vi "JV Measurement.vi"(9 "Max (V)":dbl=1.4, 11 "Step (V)":dbl=0.01) -> ()   [LabVIEW 2011]
uses:
  <instrlib>/keithley_24xx/Keithley 24XX/Public/Data/Read (Single Point).vi
  <instrlib>/keithley_24xx/Keithley 24XX/Keithley 24XX.lvlib
panel:
  in  "Variable Value":string="x"
  in  "Variable":string="x"
  in  "Tab Control":enum32{"J-V Scan", "J-t Scan"}(tab)
  in  "Min (V)":dbl
  in  "Stabilisation mode":enum16{"Voltage", "Current"}(ring)
  in  "Stabilisation time (s)":dbl=5.0
  in  "Stabilisation level \n(A or V depending on mode)":dbl=1.4
  in  "Device Area (cm^2)":dbl=0.12
  in  "Measurement Delay (ms)":dbl=10.0
  in  "Initial scan direction":bool=TRUE
  in  "Device Structure":bool
  in  "J-V Scan":bool
  in  "Exit Program":bool
  in  "Device Structure":bool
  in  "Initial scan direction":bool=TRUE
  in  "Measurement Delay (ms)":dbl=100.0
  in  "Device Area (cm^2)":dbl=0.12
  in  "Min (V)":dbl
  in  "Max (V)":dbl=1.4
  in  "Step Voltage (V)":dbl=0.1
  in  "J-t Scan":bool
  in  "Step time (s)":dbl=1.0
  in  "Integration time":enum16{"Fast", "Normal", "High Accuracy"}(ring)
  in  "Pixel":string(combo)="1"
  in  "Condition":string(combo)="Light"
  in  "Compliance  Level":dbl=0.1
  out "Log Table":string[][](table)
  out "JV Curve":cluster{"Y":dbl[], "Y":dbl[]}[](graph)
  in  "Sample Name":string
  in  "Experiment Title":string
  in  "User Name":string
  # "Label"
  # "Pixel"
  # "Condition"
  # "Jsc"
  # "Voc"
  # "PCE"
  # "FF"
  # "Vmp"
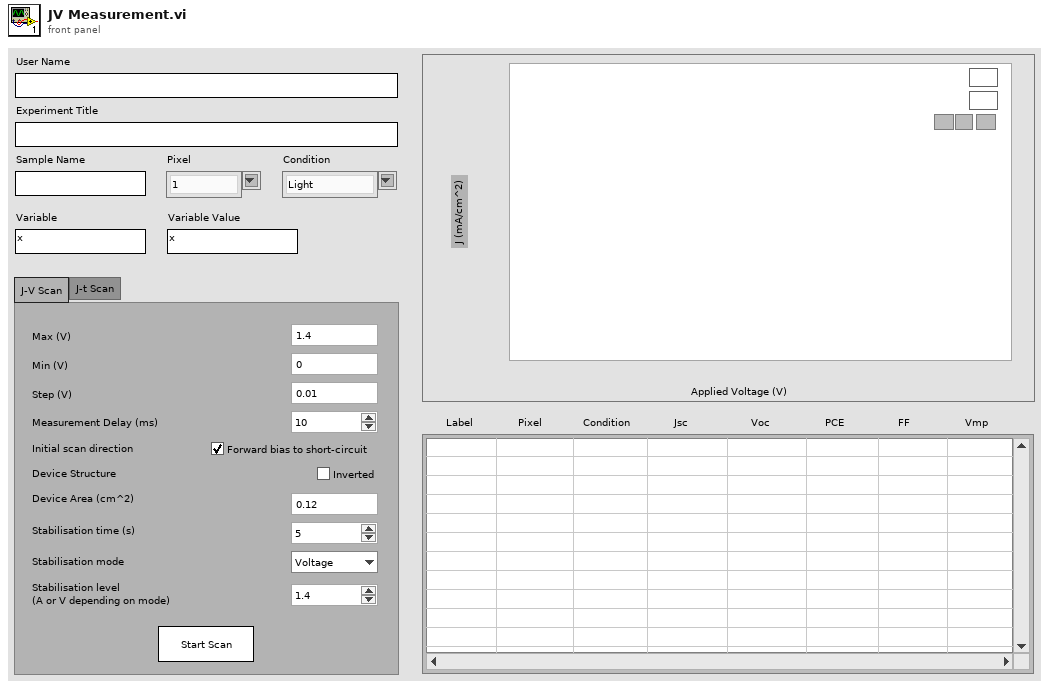
[diagram p1: front panel]
types:
  T1 = cluster{"Cell position":i32, "Cell Label":string, "Pixel":i32, "Area":dbl, "Variable":string, "Variable Value":string, "Scan settings in queue":u16, "Light or dark":string}
  T2 = typedef "imagedata.ctl" = cluster{"image type":i32, "image depth":i32, "image":u8[], "mask":u8[], "colors":u32[], "Rectangle":cluster{"left":i16, "top":i16, "right":i16, "bottom":i16}}
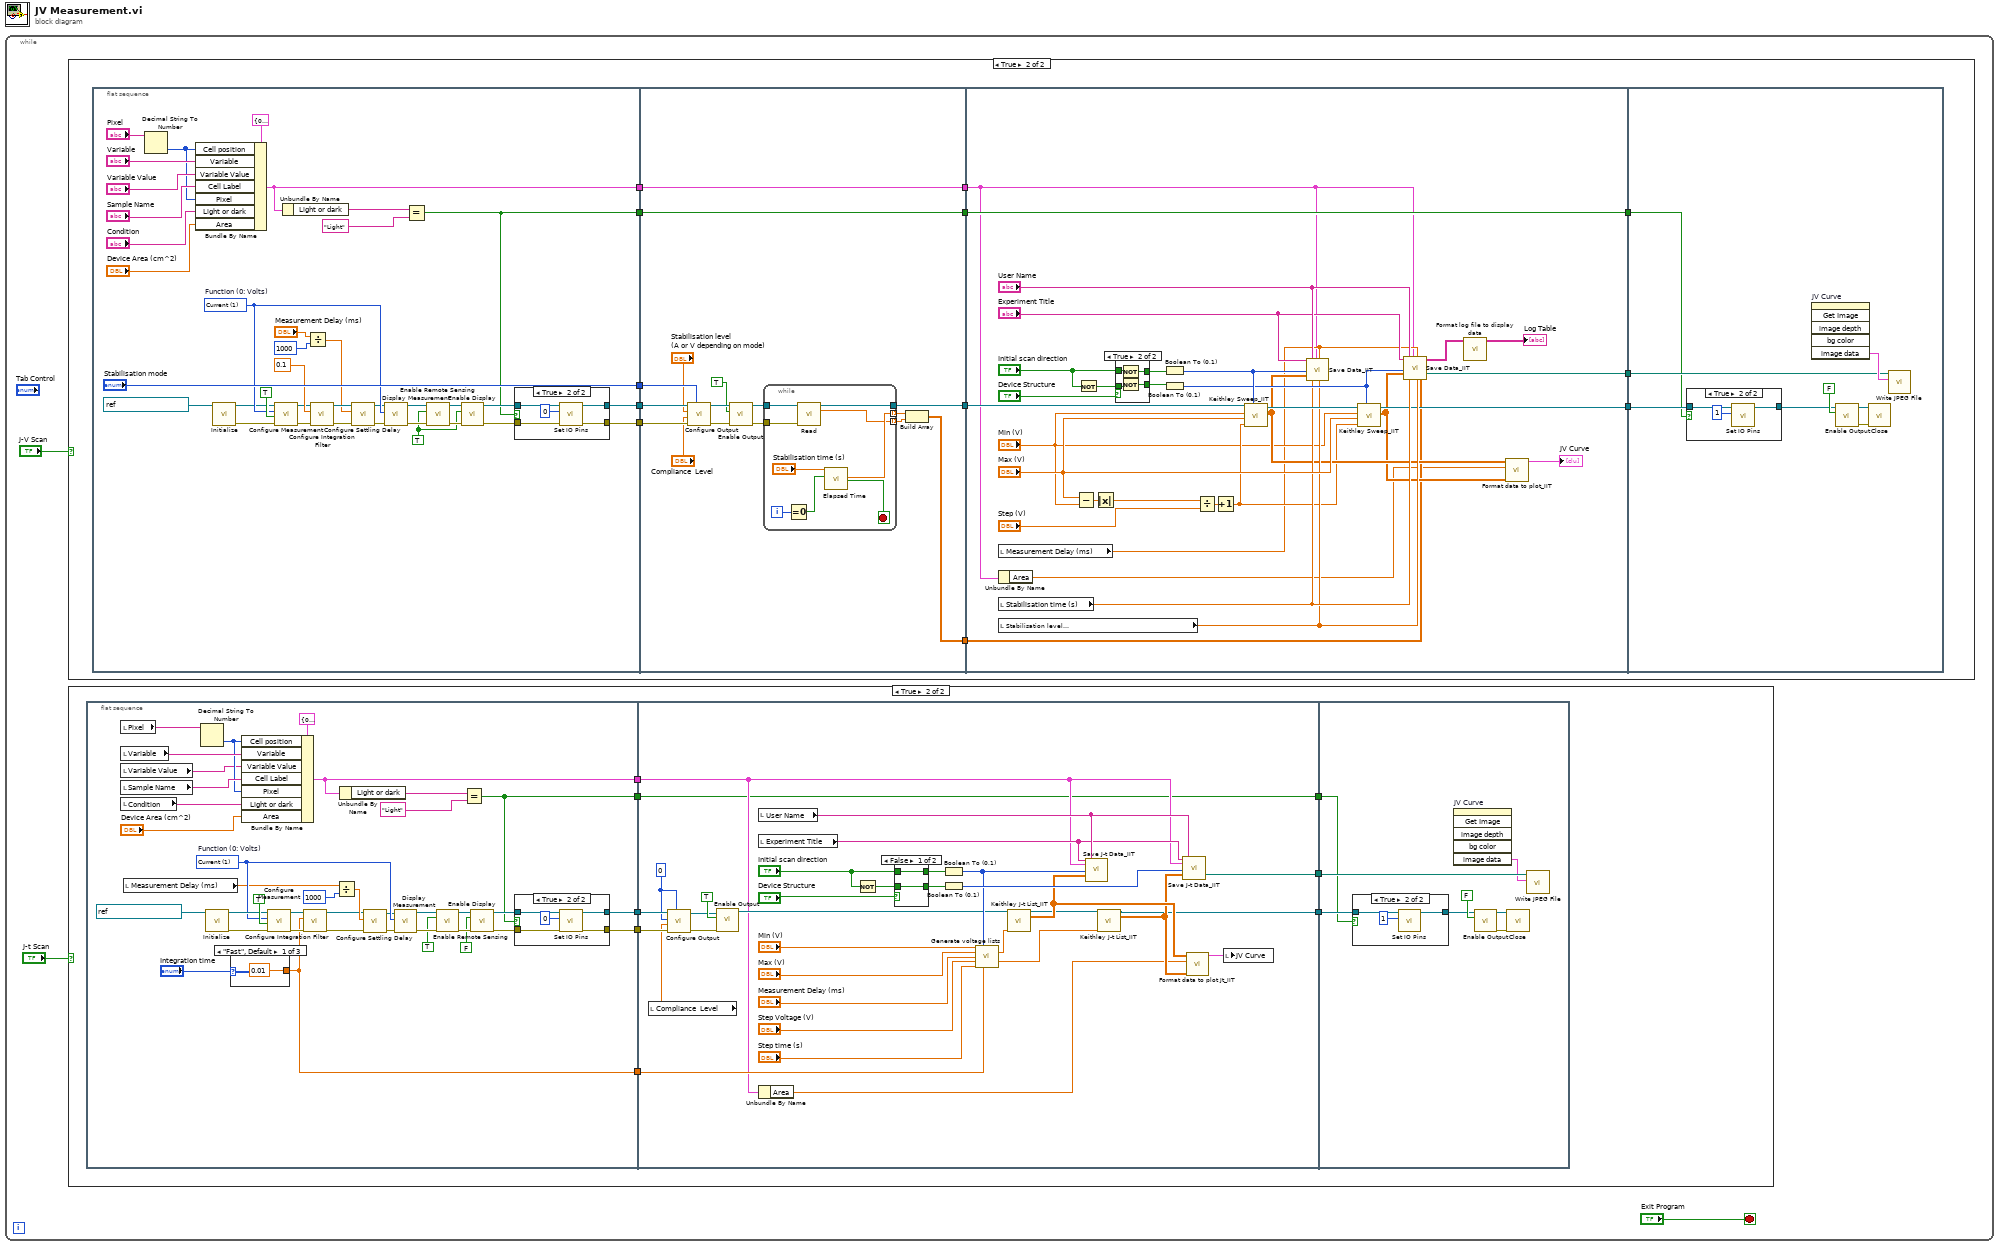
[diagram p0: block diagram]
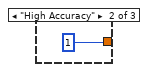
[diagram p4: hidden frame]
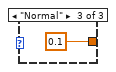
[diagram p5: hidden frame]
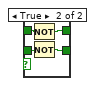
[diagram p6: hidden frame]
diagram:
  n1 = while {
    stop <- "Exit Program" stop-if-true
    n2 = case shown="True" "J-V Scan" {
      frame False {
      }
      frame True {
        n3 = flat-sequence {
          tunnel: ["Stabilisation mode"] -> w123
          tunnel: [w136] -> w122
          tunnel: [w137] -> w121
          tunnel: [w125] -> w115
          tunnel: [w124] -> w112
          tunnel: w123 -> [w179]
          tunnel: w122 -> [w180]
          tunnel: w121 -> [w181]
          tunnel: [w173] -> w120
          tunnel: [w170] -> w117
          tunnel: [w169] -> w116
          tunnel: w115 -> [w169]
          tunnel: [w168] -> w113
          tunnel: w112 -> [w168]
          tunnel: [w211] -> w119
          tunnel: [w199] -> w118
          tunnel: w120 -> [w224]
          tunnel: w117 -> [w198]
          tunnel: w116 -> [w196]
          tunnel: [w197] -> w114
          tunnel: w113 -> [w197]
          tunnel: w119 -> [w233]
          tunnel: w118 -> [w234]
          tunnel: w114 -> [w231]
          frame #0 {
            w140 = TRUE ("Enable Output (T: Enable)")
            w154 = u16 1 items=["Volts", "Current", "Resistance"]  # Function (0: Volts)
            n4 = Decimal String To Number(string="Pixel") -> (number=w129:i32)  [unwired: 2 in, 1 out]
            n5 = Bundle By Name(cluster=T1 {"Cell position"=0, "Cell Label"="", "Pixel"=0, "Area"=0.0, "Variable"="", "Variable Value"="", "Scan settings in queue"=0, "Light or dark"=""}, "Cell position"=w129, "Variable"="Variable", "Variable Value"="Variable Value", "Cell Label"="Sample Name", "Pixel"=w129, "Light or dark"="Condition", "Area"="Device Area (cm^2)") -> (w125:T1)
            n6 = call <instrlib>:"Initialize.vi"("VISA resource name"=refnum<visa-resource-name> "GPIB0::24::INSTR") -> ("error out"=w143:errorcluster, "VISA resource name out"=w144:refnum<visa-resource-name>)  [unwired: 4 in, 5 out]
            n7 = call <instrlib>:"Configure Measurement.vi"("error in (no error)"=w143, "Enable Auto Range (T:Enable)"=TRUE, "Function (0: Volts)"=w154, "VISA resource name"=w144) -> ("error out"=w146:errorcluster, "VISA resource name out"=w145:refnum<visa-resource-name>)  [unwired: 6 in]
            n8 = Unbundle By Name(w125) -> ("Light or dark"=w126:string)
            n9 = Divide(x="Measurement Delay (ms)", y=1000) -> (x/y=w153:dbl)
            n10 = call <instrlib>:"Configure Integration Filter.vi"("error in (no error)"=w146, "Measurement Speed (1 PLC)"=0.1, "VISA resource name"=w145) -> ("error out"=w156:errorcluster, "VISA resource name out"=w155:refnum<visa-resource-name>)  [unwired: 7 in]
            n11 = call <instrlib>:"Configure Settling Delay.vi"("error in (no error)"=w156, "Manual Settling Delay (0 sec)"=w153, "VISA resource name"=w155) -> ("error out"=w150:errorcluster, "VISA resource name out"=w149:refnum<visa-resource-name>)  [unwired: 7 in]
            n12 = call <instrlib>:"Display Measurement.vi"("error in (no error)"=w150, "Displayed Measurement (0: Voltage)"=w154, "VISA resource name"=w149) -> ("error out"=w148:errorcluster, "VISA resource name out"=w147:refnum<visa-resource-name>)  [unwired: 7 in]
            n13 = Equal?(x=w126, y="Light") -> (x = y?=w124:bool)
            n14 = call <instrlib>:"Enable Remote Sensing.vi"("error in (no error)"=w148, "Enable Remote Sensing (T: Enable)"=w140, "VISA resource name"=w147) -> ("error out"=w141:errorcluster, "VISA resource name out"=w142:refnum<visa-resource-name>)  [unwired: 7 in]
            n15 = call <instrlib>:"Enable Display.vi"("error in (no error)"=w141, "Enable Display (T: Enable)"=w140, "VISA resource name"=w142) -> ("error out"=w138:errorcluster, "VISA resource name out"=w139:refnum<visa-resource-name>)  [unwired: 7 in]
            n16 = case shown="True" w124 {
              tunnel: w139 -> [w162 w166]
              tunnel: w138 -> [w161 w165]
              tunnel: [w162 w164] -> w137
              tunnel: [w161 w163] -> w136
              frame False {
              }
              frame True {
                n17 = call <instrlib>:"Set IO Pins.vi"("error in (no error)"=w165, "Output Pattern (0)"=0, "VISA resource name"=w166) -> ("error out"=w163:errorcluster, "VISA resource name out"=w164:refnum<visa-resource-name>)  [unwired: 7 in]
              }
            }
          }
          frame #1 {
            n18 = call <instrlib>:"Configure Output.vi"("Source Mode  (0: Voltage)"=w179, "error in (no error)"=w180, "Compliance  Level (0.1)"="Compliance  Level", "Output Level (0)"="Stabilisation level \n(A or V depending on mode)", "VISA resource name"=w181) -> ("error out"=w183:errorcluster, "VISA resource name out"=w182:refnum<visa-resource-name>)  [unwired: 5 in]
            n19 = call <instrlib>:"Enable Output.vi"("error in (no error)"=w183, "Enable Output (T: Enable)"=TRUE ("Output (Off)"), "VISA resource name"=w182) -> ("error out"=w174:errorcluster, "VISA resource name out"=w175:refnum<visa-resource-name>)  [unwired: 7 in]
            n20 = while {
              tunnel: w175 -> [w192]
              tunnel: w174 -> [w191]
              tunnel: [w190] -> w173
              tunnel: [w187] -> w172 mode=indexing
              tunnel: [w186] -> w171 mode=indexing
              i -> [w185]
              stop <- w188 stop-if-true
              n21 = Equal To 0?(x=w185) -> (x = 0?=w184:bool)
              n22 = call-poly <instrlib>:"Read.vi"("VISA resource name"=w192, "error in (no error)"=w191) -> ("VISA resource name out"=w190:refnum<visa-resource-name>, "Current"=w186:sgl)  [unwired: 7 in, 5 out]
              n23 = call "Elapsed Time"("Time Target (s)"="Stabilisation time (s)", "Reset"=w184) -> ("Elapsed Time (s)"=w187:dbl, "Time has Elapsed"=w188:bool)  [unwired: 10 in, 6 out]
            }
            n24 = Build Array(w172, w171) -> (w170:dbl[][])
          }
          frame #2 {
            n25 = local read "Measurement Delay (ms)"() -> (w200:dbl)
            n26 = Unbundle By Name(w196) -> ("Area"=w195:dbl)
            n27 = local read "Stabilisation time (s)"() -> (w213:dbl)
            n28 = local read "Stabilisation level \n(A or V depending on mode)"() -> (w212:dbl)
            n29 = Subtract(x="Max (V)", y="Min (V)") -> (x-y=w221:dbl)
            n30 = Not(x="Initial scan direction") -> (.not. x?=w203:bool)
            n31 = Absolute Value(x=w221) -> (abs(x)=w222:dbl)
            n32 = case shown="True" "Device Structure" {
              tunnel: [w226 w230] -> w205
              tunnel: [w225 w229] -> w204
              tunnel: w203 -> [w225 w228]
              tunnel: "Initial scan direction" -> [w226 w227]
              frame False {
              }
              frame True {
                n33 = Not(x=w227) -> (.not. x?=w230:bool)
                n34 = Not(x=w228) -> (.not. x?=w229:bool)
              }
            }
            n35 = Boolean To (0,1)(Boolean=w205) -> (0, 1=w219:i16)
            n36 = Boolean To (0,1)(Boolean=w204) -> (0, 1=w214:i16)
            n37 = Divide(x=w222, y="Step (V)") -> (x/y=w208:dbl)
            n38 = Increment(x=w208) -> (x+1=w207:dbl)
            n39 = call "Keithley Sweep_IIT.vi"("Sweep Direction"=w219, "Number of Points"=w207, "Maximum Amplitude"="Max (V)", "Minimum Amplitude"="Min (V)", "VISA resource name out 2"=w224) -> ("Data Array"=w210:dbl[][], "VISA resource name out"=w218:refnum<visa-resource-name>)  [unwired: 2 in, 1 out]
            n40 = call "Save Data_IIT.vi"("Experiment Indicator"="Experiment Title", "Scan direction"=w219, "Data Array"=w210, "Username"="User Name", "Stabilisation time (ms)"=w213, "Cell details cluster"=w196, "Measurement Delay (ms)"=w200, "Stabilisation level \n(A or V depending on mode)"=w212) -> ()  [unwired: 8 in, 4 out]
            n41 = call "Keithley Sweep_IIT.vi"("Sweep Direction"=w214, "Number of Points"=w207, "Maximum Amplitude"="Max (V)", "Minimum Amplitude"="Min (V)", "VISA resource name out 2"=w218) -> ("Data Array"=w209:dbl[][], "VISA resource name out"=w211:refnum<visa-resource-name>)  [unwired: 2 in, 1 out]
            n42 = call "Save Data_IIT.vi"("Experiment Indicator"="Experiment Title", "Scan direction"=w214, "Data Array"=w209, "Username"="User Name", "Stabilisation time (ms)"=w213, "Cell details cluster"=w196, "Measurement Delay (ms)"=w200, "Stabilisation level \n(A or V depending on mode)"=w212, "Stabilisation Data"=w198) -> ("Master Log"=w194:string[][], "File path for JV image"=w199:path)  [unwired: 7 in, 2 out]
            n43 = call "Format log file to display data.vi"("Master Log"=w194) -> ("Formatted table"=→"Log Table":string[][])  [unwired: 10 in]
            n44 = call "Format data to plot_IIT.vi"("Data Array 2"=w209, "Device Area (cm^2)"=w195, "Data Array"=w210) -> ("JV Curve"=→"JV Curve":cluster{"Y":dbl[], "Y":dbl[]}[])  [unwired: 8 in]
          }
          frame #3 {
            n45 = case shown="True" w231 {
              tunnel: w233 -> [w239 w241]
              tunnel: [w239 w240] -> w232
              frame False {
              }
              frame True {
                n46 = call <instrlib>:"Set IO Pins.vi"("Output Pattern (0)"=1, "VISA resource name"=w241) -> ("VISA resource name out"=w240:refnum<visa-resource-name>)  [unwired: 8 in, 1 out]
              }
            }
            n47 = invoke on="JV Curve" class="XYGraph (strict)" method="Get Image"() -> ("image data"=w235:T2)  [unwired: 6 in, 5 out]
            n48 = call <instrlib>:"Enable Output.vi"("Enable Output (T: Enable)"=FALSE ("Output (Off)"), "VISA resource name"=w232) -> ("error out"=w237:errorcluster, "VISA resource name out"=w238:refnum<visa-resource-name>)  [unwired: 8 in]
            n49 = call <instrlib>:"Close.vi"("error in (no error)"=w237, "VISA resource name"=w238) -> ()  [unwired: 9 in, 1 out]
            n50 = call <vilib>:"Write JPEG File.vi"("image data"=w235, "path to JPEG file"=w234) -> ()  [unwired: 8 in, 2 out]
          }
        }
      }
    }
    n51 = case shown="True" "J-t Scan" {
      frame False {
      }
      frame True {
        n52 = flat-sequence {
          tunnel: [w14] -> w11
          tunnel: [w15] -> w10
          tunnel: [w28] -> w7
          tunnel: [w13] -> w6
          tunnel: [w12] -> w4
          tunnel: [w63] -> w9
          tunnel: [w90] -> w8
          tunnel: w10 -> [w82]
          tunnel: w11 -> [w81]
          tunnel: w7 -> [w70]
          tunnel: w6 -> [w62]
          tunnel: [w60] -> w5
          tunnel: w4 -> [w60]
          tunnel: w9 -> [w102]
          tunnel: w8 -> [w104]
          tunnel: w5 -> [w100]
          frame #0 {
            w38 = u16 1 items=["Volts", "Current", "Resistance"]  # Function (0: Volts)
            n53 = local read "Pixel"() -> (w26:string)
            n54 = local read "Variable"() -> (w25:string)
            n55 = local read "Variable Value"() -> (w20:string)
            n56 = local read "Sample Name"() -> (w24:string)
            n57 = local read "Condition"() -> (w22:string)
            n58 = local read "Measurement Delay (ms)"() -> (w30:dbl)
            n59 = Decimal String To Number(string=w26) -> (number=w23:i32)  [unwired: 2 in, 1 out]
            n60 = call <instrlib>:"Initialize.vi"("VISA resource name"=refnum<visa-resource-name> "GPIB0::24::INSTR") -> ("error out"=w42:errorcluster, "VISA resource name out"=w43:refnum<visa-resource-name>)  [unwired: 4 in, 5 out]
            n61 = case shown="\"Fast\", Default" "Integration time" {
              tunnel: [0.01 1 0.1] -> w28
              frame "Fast", Default {
              }
              frame "High Accuracy" {
              }
              frame "Normal" {
              }
            }
            n62 = Bundle By Name(cluster=T1 {"Cell position"=0, "Cell Label"="", "Pixel"=0, "Area"=0.0, "Variable"="", "Variable Value"="", "Scan settings in queue"=0, "Light or dark"=""}, "Cell position"=w23, "Variable"=w25, "Variable Value"=w20, "Cell Label"=w24, "Pixel"=w23, "Light or dark"=w22, "Area"="Device Area (cm^2)") -> (w13:T1)
            n63 = call <instrlib>:"Configure Measurement.vi"("error in (no error)"=w42, "Enable Auto Range (T:Enable)"=TRUE, "Function (0: Volts)"=w38, "VISA resource name"=w43) -> ("error out"=w45:errorcluster, "VISA resource name out"=w44:refnum<visa-resource-name>)  [unwired: 6 in]
            n64 = call <instrlib>:"Configure Integration Filter.vi"("error in (no error)"=w45, "Measurement Speed (1 PLC)"=w28, "VISA resource name"=w44) -> ("error out"=w31:errorcluster, "VISA resource name out"=w34:refnum<visa-resource-name>)  [unwired: 7 in]
            n65 = Divide(x=w30, y=1000) -> (x/y=w36:dbl)
            n66 = Unbundle By Name(w13) -> ("Light or dark"=w18:string)
            n67 = call <instrlib>:"Configure Settling Delay.vi"("error in (no error)"=w31, "Manual Settling Delay (0 sec)"=w36, "VISA resource name"=w34) -> ("error out"=w32:errorcluster, "VISA resource name out"=w33:refnum<visa-resource-name>)  [unwired: 7 in]
            n68 = call <instrlib>:"Display Measurement.vi"("error in (no error)"=w32, "Displayed Measurement (0: Voltage)"=w38, "VISA resource name"=w33) -> ("error out"=w47:errorcluster, "VISA resource name out"=w46:refnum<visa-resource-name>)  [unwired: 7 in]
            n69 = call <instrlib>:"Enable Remote Sensing.vi"("error in (no error)"=w47, "Enable Remote Sensing (T: Enable)"=TRUE ("Enable Output (T: Enable)"), "VISA resource name"=w46) -> ("error out"=w40:errorcluster, "VISA resource name out"=w41:refnum<visa-resource-name>)  [unwired: 7 in]
            n70 = Equal?(x=w18, y="Light") -> (x = y?=w12:bool)
            n71 = call <instrlib>:"Enable Display.vi"("error in (no error)"=w40, "Enable Display (T: Enable)"=FALSE ("Enable Output (T: Enable)"), "VISA resource name"=w41) -> ("error out"=w16:errorcluster, "VISA resource name out"=w17:refnum<visa-resource-name>)  [unwired: 7 in]
            n72 = case shown="True" w12 {
              tunnel: w17 -> [w51 w55]
              tunnel: w16 -> [w50 w54]
              tunnel: [w51 w53] -> w15
              tunnel: [w50 w52] -> w14
              frame False {
              }
              frame True {
                n73 = call <instrlib>:"Set IO Pins.vi"("error in (no error)"=w54, "Output Pattern (0)"=0, "VISA resource name"=w55) -> ("error out"=w52:errorcluster, "VISA resource name out"=w53:refnum<visa-resource-name>)  [unwired: 7 in]
              }
            }
          }
          frame #1 {
            w78 = 0
            n74 = local read "Compliance  Level"() -> (w77:dbl)
            n75 = call <instrlib>:"Configure Output.vi"("Source Mode  (0: Voltage)"=w78, "error in (no error)"=w81, "Compliance  Level (0.1)"=w77, "Output Level (0)"=w78, "VISA resource name"=w82) -> ("error out"=w79:errorcluster, "VISA resource name out"=w80:refnum<visa-resource-name>)  [unwired: 5 in]
            n76 = call <instrlib>:"Enable Output.vi"("error in (no error)"=w79, "Enable Output (T: Enable)"=TRUE ("Output (Off)"), "VISA resource name"=w80) -> ("VISA resource name out"=w69:refnum<visa-resource-name>)  [unwired: 7 in, 1 out]
            n77 = local read "User Name"() -> (w88:string)
            n78 = local read "Experiment Title"() -> (w87:string)
            n79 = Unbundle By Name(w62) -> ("Area"=w61:dbl)
            n80 = Not(x="Initial scan direction") -> (.not. x?=w91:bool)
            n81 = case shown="False" "Device Structure" {
              tunnel: [w95 w99] -> w93
              tunnel: [w94 w98] -> w92
              tunnel: w91 -> [w94 w97]
              tunnel: "Initial scan direction" -> [w95 w96]
              frame False {
              }
              frame True {
                n82 = Not(x=w96) -> (.not. x?=w99:bool)
                n83 = Not(x=w97) -> (.not. x?=w98:bool)
              }
            }
            n84 = Boolean To (0,1)(Boolean=w93) -> (0, 1=w76:i16)
            n85 = Boolean To (0,1)(Boolean=w92) -> (0, 1=w83:i16)
            n86 = call "Generate voltage lists.vi"("MinVoltage"="Min (V)", "Initial sweep direction"=w76, "Max Voltage"="Max (V)", "Measurement Delay (ms)"="Measurement Delay (ms)", "V step"="Step Voltage (V)", "t step"="Step time (s)", "NPLC"=w70) -> ("Voltage Forward List"=w68:dbl[], "Voltage Reverse List"=w65:dbl[])  [unwired: 7 in]
            n87 = call "Keithley J-t List_IIT.vi"("VISA resource name in"=w69, "Voltage List"=w68) -> ("VISA resource name out"=w66:refnum<visa-resource-name>, "Data Array"=w67:dbl[][])  [unwired: 11 in, 1 out]
            n88 = call "Save J-t Data_IIT.vi"("Experiment Indicator"=w87, "Cell details cluster"=w62, "Scan direction"=w76, "Data Array"=w67, "Username"=w88) -> ()  [unwired: 13 in, 2 out]
            n89 = call "Keithley J-t List_IIT.vi"("VISA resource name in"=w66, "Voltage List"=w65) -> ("VISA resource name out"=w63:refnum<visa-resource-name>, "Data Array"=w64:dbl[][])  [unwired: 11 in, 1 out]
            n90 = call "Save J-t Data_IIT.vi"("Experiment Indicator"=w87, "Cell details cluster"=w62, "Scan direction"=w83, "Data Array"=w64, "Username"=w88) -> ("File path for JV image"=w90:path)  [unwired: 13 in, 1 out]
            n91 = call "Format data to plot Jt_IIT.vi"("Data Array 2"=w64, "Device Area (cm^2)"=w61, "Data Array"=w67) -> ("JV Curve"=w89:cluster{"Y":dbl[], "Y":dbl[]}[])  [unwired: 8 in]
            n92 = local write "JV Curve"(w89) -> ()
          }
          frame #2 {
            n93 = case shown="True" w100 {
              tunnel: w102 -> [w108 w110]
              tunnel: [w108 w109] -> w101
              frame False {
              }
              frame True {
                n94 = call <instrlib>:"Set IO Pins.vi"("Output Pattern (0)"=1, "VISA resource name"=w110) -> ("VISA resource name out"=w109:refnum<visa-resource-name>)  [unwired: 8 in, 1 out]
              }
            }
            n95 = invoke on="JV Curve" class="XYGraph (strict)" method="Get Image"() -> ("image data"=w103:T2)  [unwired: 6 in, 5 out]
            n96 = call <instrlib>:"Enable Output.vi"("Enable Output (T: Enable)"=FALSE ("Output (Off)"), "VISA resource name"=w101) -> ("error out"=w106:errorcluster, "VISA resource name out"=w107:refnum<visa-resource-name>)  [unwired: 8 in]
            n97 = call <instrlib>:"Close.vi"("error in (no error)"=w106, "VISA resource name"=w107) -> ()  [unwired: 9 in, 1 out]
            n98 = call <vilib>:"Write JPEG File.vi"("image data"=w103, "path to JPEG file"=w104) -> ()  [unwired: 8 in, 2 out]
          }
        }
      }
    }
  }
